vi "Acquire Data.vi"(6 "Data Encoding Width (3 Byte)":u16(ring)=3 items=["2 Byte"=2, "3 Byte"=3], 7 "Cluster Count (1)":dbl=1.0, 8 "error in (no error)":errorcluster, 9 "End Point (120°)":dbl=120.0, 10 "Start Point (-120°)":dbl=-120.0, 11 "VISA resource name":refnum<visa-resource-name>) -> (0 "error out":errorcluster, 1 "Direction":dbl[](array[numeric]), 2 "Magnitude":dbl[](array[numeric]), 3 "VISA resource name out":refnum<visa-resource-name>)   [LabVIEW 2014, in "Hokuyo URG Series.lvlib"]
doc: "This VI takes three parameters (start point, end point, cluster count) and returns two arrays which describe the magnitude and angle at which the data was acquired. \n\nThe reference for the angles (in the Direction array) is the center of the device which is 0° with positive angles to the left of center and negative angles to the right.\n\nThe URG-04LX can take measurements in the range of -120° to 120° and has an \"operating range\" of -135° to 135°. \n\nCluster Count refers to the number of measurements which are clustered together. \n<b>Ex:</b>If the cluster count is 3 then the smallest of three measurements is returned.\n\nThe Magnitude array is associated with the Direction array. \n<b>Ex:</b> If the information for the first measurement is desired, then the 0th index of each array is accessed and returns the magnitude and direction of the first measurement.\n\nIf checksums are being used and the checksum fails, the data returned in the magnitude array will default to -1."
uses:
  Hokuyo URG Series.lvlib
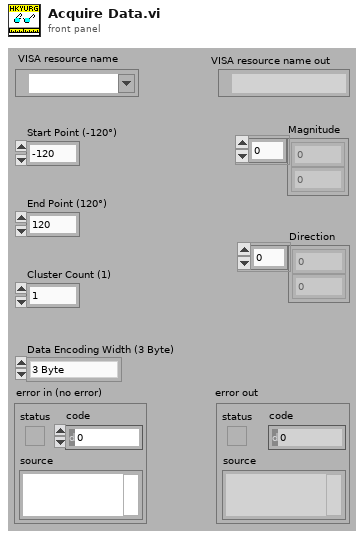
[diagram p1: front panel]
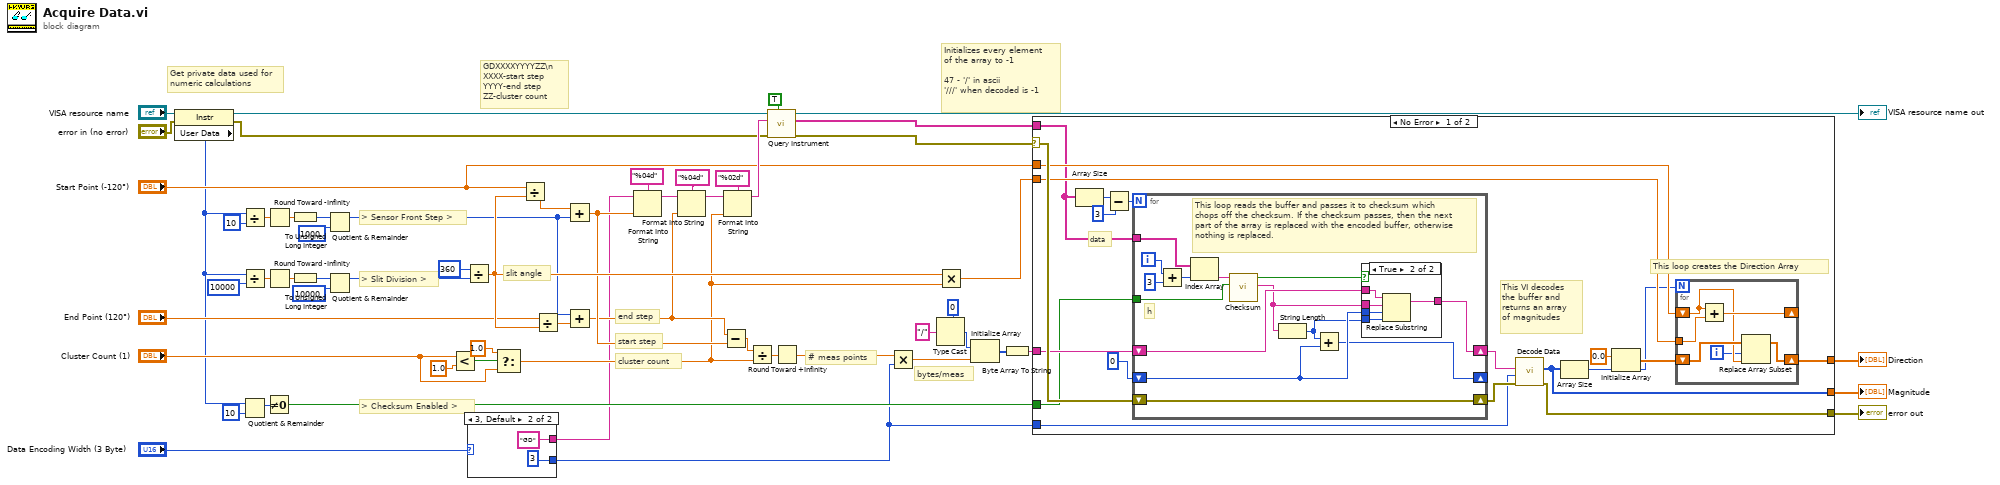
[diagram p0: block diagram]
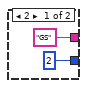
[diagram p2: hidden frame]
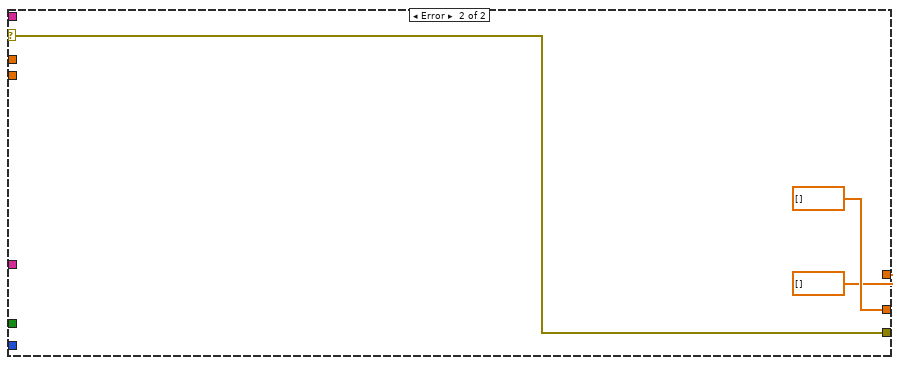
[diagram p4: hidden frame]
diagram:
  # "Get private data used for numeric calculations"
  # "> Slit Division >"
  # "> Sensor Front Step >"
  # "> Checksum Enabled >"
  # "bytes/meas"
  # "# meas points"
  # "cluster count"
  # "start step"
  # "end step"
  # "slit angle"
  # "Initializes every element\nof the array to -1\n\n47 - '/' in ascii\n'///' when decoded is -1"
  # "GDXXXXYYYYZZ\\n\nXXXX-start step\nYYYY-end step\nZZ-cluster count"
  n1 = property class="Instr"(reference="VISA resource name", error in="error in (no error)") -> (reference out=w9:refnum<visa-resource-name>, error out=w8:errorcluster, "User Data"=w11:u32)
  n2 = Divide(x=w11, y=u32 10) -> (x/y=w24:dbl)
  n3 = Divide(x=w11, y=u32 10000) -> (x/y=w18:dbl)
  n4 = Quotient & Remainder(x=w11, y=u32 10) -> (x-y*floor(x/y)=w26:u32)  [unwired: 1 out]
  n5 = Not Equal To 0?(x=w26) -> (x != 0?=w25:bool)
  n6 = Round Toward -Infinity(1:w24) -> (0:w20:dbl)
  n7 = Round Toward -Infinity(1:w18) -> (0:w17:dbl)
  n8 = To Unsigned Long Integer(number=w20) -> (unsigned 32bit integer=w23:u32)
  n9 = To Unsigned Long Integer(number=w17) -> (unsigned 32bit integer=w16:u32)
  n10 = Quotient & Remainder(x=w23, y=u32 1000) -> (x-y*floor(x/y)=w22:u32)  [unwired: 1 out]
  n11 = Quotient & Remainder(x=w16, y=u32 10000) -> (x-y*floor(x/y)=w14:u32)  [unwired: 1 out]
  n12 = Less?(x="Cluster Count (1)", y=1.0) -> (x < y?=w43:bool)
  n13 = Divide(x=u32 360 ("y"), y=w14) -> (x/y=w38:dbl)
  n14 = case shown="3, Default" "Data Encoding Width (3 Byte)" {
    tunnel: ["GS" ("initial string") "GD" ("initial string")] -> w4
    tunnel: [2 ("byte encoding width") 3 ("byte encoding width")] -> w3
    frame 2 {
    }
    frame 3, Default {
    }
  }
  n15 = Select(t=1.0, s=w43, f="Cluster Count (1)") -> (s? t:f=w30:dbl)
  n16 = Divide(x="Start Point (-120°)", y=w38) -> (x/y=w36:dbl)
  n17 = Divide(x="End Point (120°)", y=w38) -> (x/y=w33:dbl)
  n18 = Add(x=w36, y=w22) -> (x+y=w35:dbl)
  n19 = Add(x=w22, y=w33) -> (x+y=w32:dbl)
  n20 = Format Into String(format string="%04d", initial string=w4, w35) -> (resulting string=w54:string)  [unwired: 1 in, 1 out]
  n21 = Format Into String(format string="%04d", initial string=w54, w32) -> (resulting string=w52:string)  [unwired: 1 in, 1 out]
  n22 = Subtract(x=w32, y=w35) -> (x-y=w48:dbl)
  n23 = Format Into String(format string="%02d", initial string=w52, w30) -> (resulting string=w51:string)  [unwired: 1 in, 1 out]
  n24 = Divide(x=w48, y=w30) -> (x/y=w49:dbl)
  n25 = call "Query Instrument.vi"("Error Query (Enabled)"=TRUE, "error in"=w8, "Command"=w51, "VISA Resource Name"=w9) -> ("error out"=w5:errorcluster, "Response Strings"=w2:string[], "VISA Resource Name Out"=→"VISA resource name out":refnum<visa-resource-name>)  [unwired: 5 in]
  n26 = Round Toward +Infinity(x=w49) -> (ceil(x): smallest int >= x=w46:dbl)
  n27 = Multiply(x=w46, y=w3) -> (x*y=w45:dbl)
  n28 = Type Cast(type=u8 0, x="/") -> (*(type *) &x=w27:u8)
  n29 = Multiply(x=w38, y=w30) -> (x*y=w50:dbl)
  n30 = Initialize Array(w27, w45) -> (w47:u8[])
  n31 = Byte Array To String(unsigned byte array=w47) -> (string=w41:string)
  n32 = case shown="No Error" w5 {
    selector: w5 -> [w82 w111]
    tunnel: [w70 w111] -> w57
    tunnel: "Start Point (-120°)" -> [w81 _]
    tunnel: w50 -> [w80 _]
    tunnel: [w75 dbl[] []] -> w59
    tunnel: [w79 dbl[] []] -> w58
    tunnel: w41 -> [w78 _]
    tunnel: w25 -> [w69 _]
    tunnel: w2 -> [w64 _]
    tunnel: w3 -> [w65 _]
    frame No Error {
      # "data"
      # "This loop creates the Direction Array"
      # "This VI decodes the buffer and returns an array of magnitudes"
      n33 = Array Size(array=w64) -> (size(s)=w68:i32)
      n34 = Subtract(x=w68, y=3) -> (x-y=w67:i32)
      n35 = for {
        N: w67 -> [_]
        shift-right: [w83] -> w76
        shift-left: w82 -> [w83]
        shift-right: [w96] -> w77
        shift-left: w78 -> [w95]
        shift-right: [w93] -> _
        shift-left: 0 -> [w94]
        tunnel: w69 -> [w91]
        tunnel: w64 -> [w90]
        i -> [w88]
        # "h"
        # "This loop reads the buffer and passes it to checksum which chops off the checksum. If the checksum passes, then the next part of the array is replaced with the encoded buffer, otherwise nothing is replaced."
        n36 = Add(x=w88, y=3) -> (x+y=w89:i32)
        n37 = Index Array(array=w90, index=w89) -> (element=w86:string)
        n38 = call "Checksum.vi"("Checksum (Off)"=w91, "Input"=w86) -> ("Data Buffer"=w85:string, "Checksum Pass?"=w92:bool)  [unwired: 8 out]
        n39 = String Length(string=w85) -> (length=w84:i32)
        n40 = Add(x=w84, y=w94) -> (x+y=w93:i32)
        n41 = case shown="True" w92 {
          tunnel: [w97 w98] -> w96
          tunnel: w95 -> [w97 w102]
          tunnel: w85 -> [_ w101]
          tunnel: w94 -> [_ w100]
          tunnel: w84 -> [_ w99]
          frame False {
          }
          frame True {
            n42 = Replace Substring(2:w99, 3:w100, 4:w101, 5:w102) -> (1:w98:string)  [unwired: 1 out]
          }
        }
      }
      n43 = call "Decode Data.vi"("error in (no error)"=w76, "n character encoding"=w65, "Input Buffer"=w77) -> ("error out"=w70:errorcluster, "Decoded Measurements"=w75:i32[])  [unwired: 2 in, 5 out]
      n44 = Array Size(array=w75) -> (size(s)=w72:i32)
      n45 = Initialize Array(0.0 ("element"), w72) -> (w73:dbl[])
      n46 = for {
        N: w72 -> [_]
        shift-right: [w107] -> _
        shift-left: w81 -> [w104]
        tunnel: w80 -> [w108]
        shift-right: [w105] -> w79
        shift-left: w73 -> [w106]
        i -> [w103]
        n47 = Add(x=w104, y=w108) -> (x+y=w107:dbl)
        n48 = Replace Array Subset(array=w106, new element=w104, index=w103) -> (w105:dbl[])
      }
    }
    frame Error {
    }
  }
  "Magnitude" <- w59
  "Direction" <- w58
  "error out" <- w57
